vi "2021_day4_task1,2.vi"() -> ()   [LabVIEW 2021]
panel:
  out "TASK2: Winning Score (Last board)":u32
  out "TASK1: Winning Score":u32
  out "Number of Drawns":i32[](array[numeric])
  out "Winning Scores":u32[](array[numeric])
  out "5x5 Bingo numbers":i32[][][](array[numeric])
  out "array":string[](array[string])
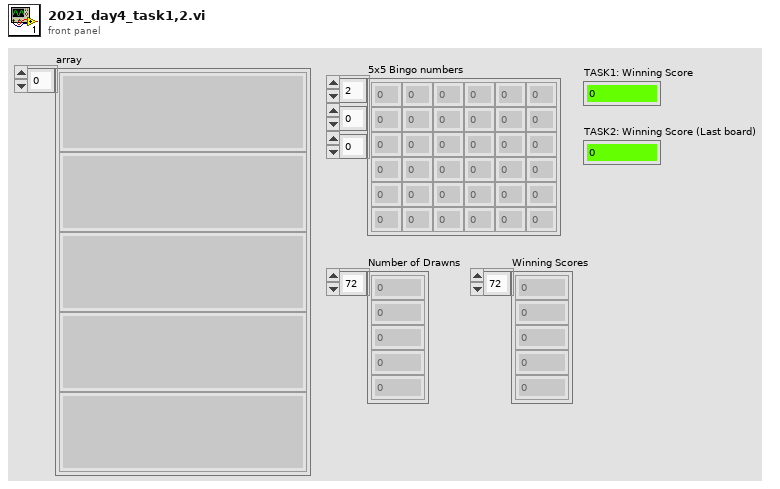
[diagram p1: front panel]
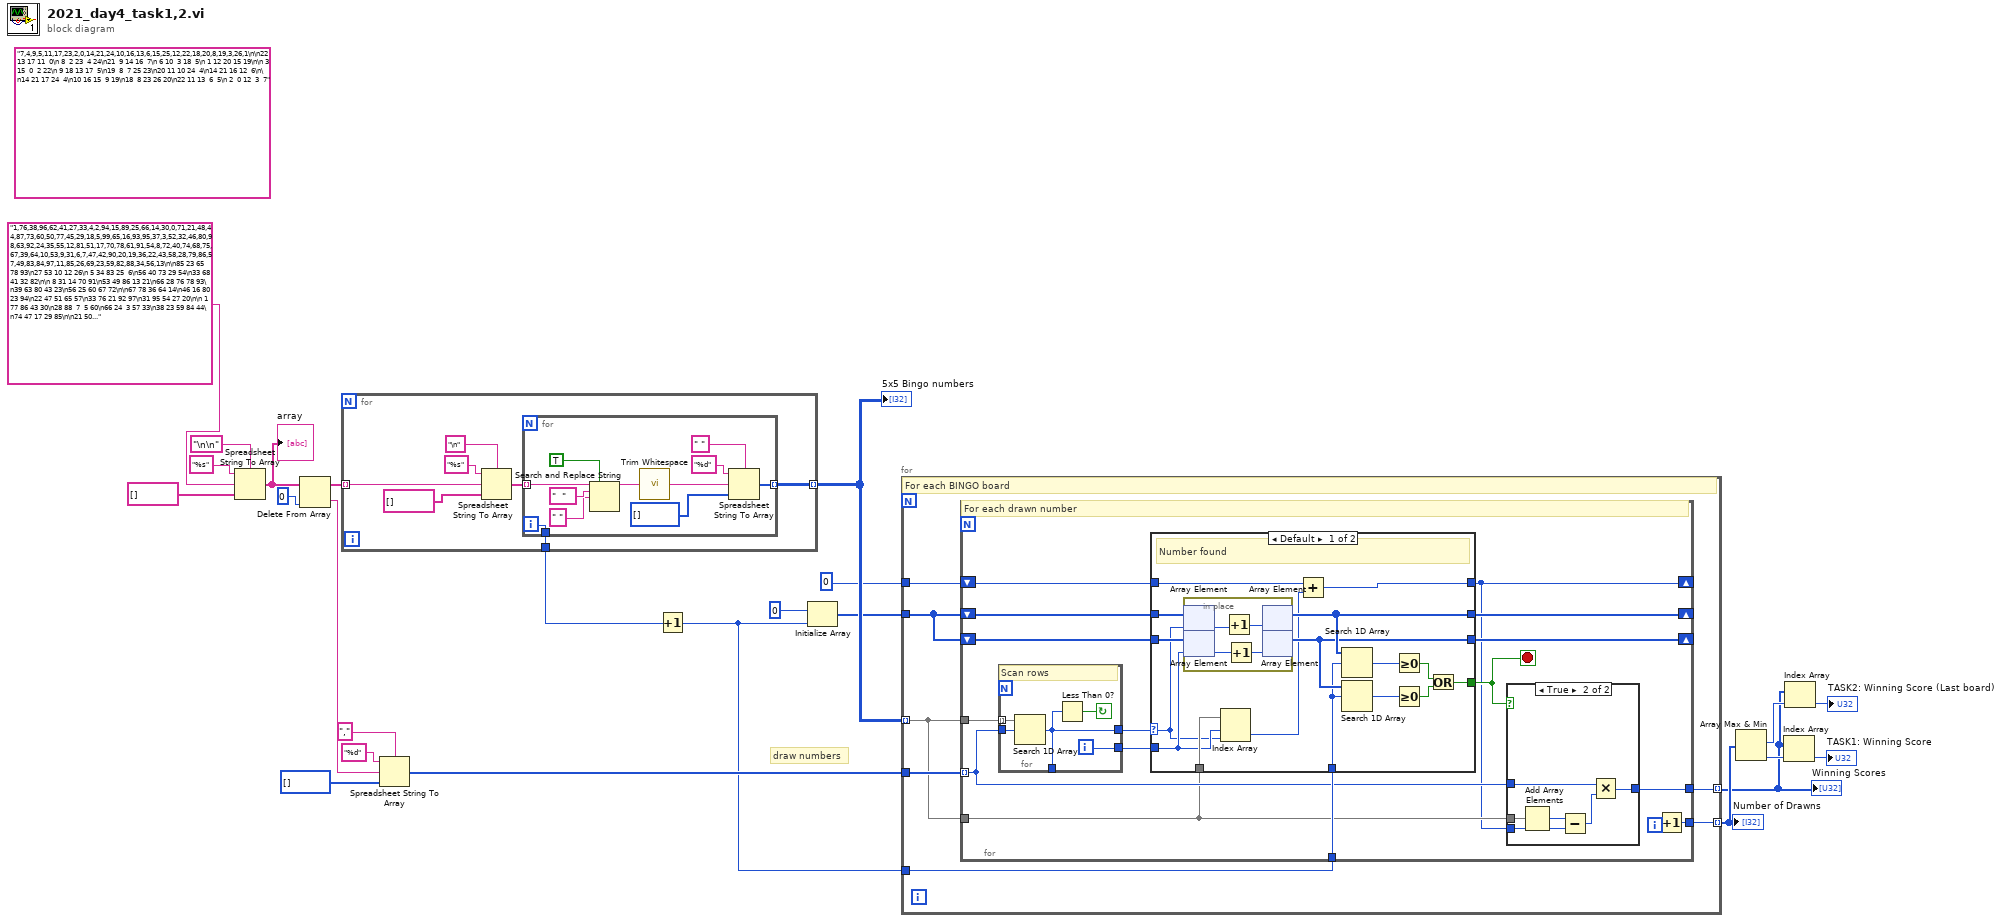
[diagram p0: block diagram]
diagram:
  (unwired) "7,4,9,5,11,17,23,2,0,14,21,24,10,16,13,6,15,25,12,22,18,20,8,19,3,26,1\n\n22 13 17 11  0\n 8  2 23  4 24\n21  9 14 16  7\n 6 10  3 18  5\n 1 12 20 15 19\n\n 3 15  0  2 22\n 9 18 13 17  5\n19  8  7 25 23\n20 11 10 24  4\n14 21 16 12  6\n\n14 21 17 24  4\n10 16 15  9 19\n18  8 23 26 20\n22 11 13  6  5\n 2  0 12  3  7"
  # "draw numbers"
  n1 = Spreadsheet String To Array(delimiter (Tab)="\n\n", format string="%s", spreadsheet string="1,76,38,96,62,41,27,33,4,2,94,15,89,25,66,14,30,0,71,21,48,44,87,73,60,50,77,45,29,18,5,99,65,16,93,95,37,3,52,32,46,80,98,63,92,24,35,55,12,81,51,17,70,78,61,91,54,8,72,40,74,68,75,67,39,64,10,53,9,31,6,7,47,42,90,20,19,36,22,43,58,28,79,86,57,49,83,84,97,11,85,26,69,23,59,82,88,34,56,13\n\n85 23 65 78 93\n27 53 10 12 26\n 5 34 83 25  6\n56 40 73 29 54\n33 68 41 32 82\n\n 8 31 14 70 91\n53 49 86 13 21\n66 28 76 78 93\n39 63 80 43 23\n56 25 60 67 72\n\n67 78 36 64 14\n46 16 80 23 94\n22 47 51 65 57\n33 76 21 92 97\n31 95 54 27 20\n\n 1 77 86 43 30\n28 88  7  5 60\n66 24  3 57 33\n38 23 59 84 44\n74 47 17 29 85\n\n21 50 86  2 70\n85 19 22 93 25\n99 38 74 30 65\n81  0 47 78 63\n34 11 51 88 64\n\n45 15 29 81 30\n75 21 88 91 49\n39 20  4 17 78\n10 12 38 11  7\n98  6 65 69 86\n\n36 20 31 44 69\n30 65 55 88 64\n74 85 82 61  5\n57 17 90 43 54\n58 83 52 23  7\n\n42 16 82 86 76\n60 26 27 59 55\n 7 53 22 78  5\n18 61 10 15 17\n28 46 14 87 77\n\n21 43 15 47 61\n24 76 28  3 27\n19 62 69 82 93\n49 29 97 74 41\n92 36 37 99 40\n\n31  4  3 62 51\n24 57 78 67 53\n13  5 76 38 55\n79  9 75 98 71\n65  1 39 18 47\n\n59  4 38 95 99\n85 68 69 93 43\n83 57 48 42 15\n47 50 80 79 90\n56 87 78 64 25\n\n21 37 14 67 95\n88 39 26 38 49\n89 83 54 77 96\n48 86 94 19 20\n43 41  8 74 58\n\n 1 36 12 90 91\n63 21 98 82 66\n39 86  7 52 77\n80 81 44 33 58\n78 30 11 51 28\n\n81 74  7 33 96\n75 60 87 47 91\n39 73 30 50 13\n 4 41  9 43 77\n34 82 72 48 12\n\n93 63 74 25 57\n29 76  9 45 70\n98 77 71 16 41\n47 54 18 14 55\n31 89 67 87 83\n\n 8 72 45 93 68\n74 26 69 94 65\n28  9 20 47 41\n46 54 21 56 22\n84 62 18 15 48\n\n20 51 81 40 69\n71 10 13 93 75\n44 86  0 95 37\n99 39 76 80 66\n14 64 49 62 27\n\n75  7 51 86 79\n43 30 61 39 16\n85 63 90 28 96\n88 78 72 31 73\n98 87 23 19 58\n\n20 95 47 97 12\n92 25 68 87 91\n37 10 78 23 63\n74 93 58 39  5\n76 51 48 72 16\n\n37 18 32 34 85\n22 31 98 42 19\n29 72 48 76 25\n47  1 21  7 53\n79 82 86 52 78\n\n20 16 47 78 92\n88 15 71 67  2\n 5 52 90 70  9\n22 49 28 82 27\n 6 19 61 73 48\n\n71 26  7 11 79\n52 30 47  1 31\n17 75 94 91 28\n81 98 23 55 21\n77 15 39 24 16\n\n 5 75 44 88 65\n89 45 23 69 19\n41 61 67 52 54\n47 38 57 12 98\n62 70 26 87 53\n\n50  4 65 77 25\n 6 21  5 27 92\n39 63 97 75 79\n60 34 87 26 74\n99 24 44 85  2\n\n13 64 38 78 21\n74 17 83 57 94\n25 39 69 53  4\n54 33 81 50 76\n42 75 19 77 26\n\n63 31 70 19 39\n38 87 15 90 75\n61 98  6 29 86\n78 62 32 11 60\n55 97 13 73 82\n\n51 63 68 84 36\n12 33 37 31  8\n18 41 34 74 23\n72 39 85 48 60\n24 19 29 88  0\n\n46 51 17 23 13\n20 93 97 99 81\n57 47 33 84 44\n28 96  2 43 56\n68 36 62 15  5\n\n81 99  5 30 10\n38 62 57  8 37\n 7 86 98  3 54\n46 82 96 15 72\n83  1 75 25 50\n\n47 57 11 61 27\n53 10 31 91 98\n76 85 55 38 23\n 6 81 67 71 70\n35 29 17 50 56\n\n24 65 15  1 89\n45 60 97 23 14\n84 56 58  5 54\n 3 72 51 46 79\n67 70 78 34 77\n\n38 11 54 23  2\n33 14 10 96 63\n43  5 36 20 30\n70 53 66 71  9\n91 90 21  7 88\n\n94 44  4 86 26\n39 70 54 50 30\n55 40 12 72 71\n68  7 66 47 91\n31 24 13  1 96\n\n79 14 40 87 68\n16 32 53 46 98\n38 95 21 89 69\n62 60 19 81 33\n70 52 28 83  0\n\n62 42 38 48 64\n61 79 78 97 98\n89  7  3 29 68\n92 76 14 67  1\n41 99 72 47 60\n\n 5 75 18 42 33\n72 61 36 31 29\n19 58  1 34 94\n54 84 92 99 38\n76 68 79 53 37\n\n14 91 37  5 98\n68 29 34 76 43\n75  0 67 33 69\n81 47 58 30 93\n88 92 42 77 54\n\n64 24 28 54 53\n72 68  3 73  4\n83  6 59 66 94\n87 80 55 20 16\n13 82 74 31 70\n\n63 92 71  0 83\n98 40 50 55  2\n88  5 85 30 23\n10 75 81 58 68\n51 31 14 89  1\n\n67 93 94 54 53\n38 71 34 40 24\n31 63 30 99 75\n 4 57 86 19 70\n60 49 87 68 74\n\n56 94 79 53  7\n24 12 19  6 99\n82 51 41 46 43\n17 49 52 78 55\n75 48 61 70 87\n\n14 55 32 21 31\n88 83 23 44  4\n 1 77 45 90 85\n46 81 51 27 62\n60 24 29 18  0\n\n95 92 91 27 26\n22 43 45 64 62\n83 23 25 85 94\n84 53 72 28 20\n75 60 52 18 73\n\n95 41  7 21 32\n58 65 16 56 97\n68 25 91 83 24\n66 89 15 55  6\n 2 30 84 10 90\n\n58 86 44 19 74\n57 89 17  6 83\n77 35 60 32 13\n97 63 62 28 76\n55 31 11  0 52\n\n33 39 59 42 45\n61 50 92  9 79\n15  0 28  5 72\n91 24 21 29 87\n86 76 43 31 93\n\n63 11 86 45 85\n96 74 66 93 32\n95 30 99 23 18\n69 97 48 15  1\n42 87 47 83 80\n\n93  5 40 64  2\n44 51 15 54 83\n69 77 90 58 11\n 0 48 43 30 55\n25 72 38 73 52\n\n89 58 71 68 15\n23 65  9 36 74\n21 29 42 79 98\n55 47 33 39 28\n16 75 91 69 57\n\n13 79 12 71  2\n60 94 99 43 82\n84 89 29 91 87\n74 80 25 32 21\n70 14 68 92 11\n\n78  1 16 51 87\n58 94 59 15 43\n79 41 50 47 39\n53 37  9 28 72\n34 63 89 35 18\n\n31 67 70 42 43\n60  2 89 49 22\n56 17 81 24 74\n20 65  1 96 51\n68  7  0 38 25\n\n59 14 29 53 19\n 9  2 11 33 44\n81  6 10 47 58\n20 34 62 55 40\n71 38 69 45 78\n\n59 36 70 42 21\n 3 16 49 79 98\n74 25  8 84 19\n61 80 47 65 64\n91 62 52  9 40\n\n 1 85 63  7  2\n 0 20 61 26 77\n99 37 74 42 76\n25 94 19 78 60\n79 72 95 22 11\n\n51 21 79 76 32\n55 23 69 19 61\n71 54 94 47 92\n 5 64  6 68 16\n91 81  9 99 30\n\n61 69 82 86 68\n66 81 28 38 36\n26 29 31 11  8\n72 51 12 95 63\n18 30 88 17 32\n\n34  8 14 42 67\n66 79 65 20 52\n37 87 74 24  3\n59 54 21 32 89\n31  4 62 76 30\n\n11 93  8 92 55\n38 72 99  3 83\n12 75  0 41 46\n17 25  5 39 48\n14 18 86 29 84\n\n 6 20 41 51 48\n 5 67 30 24 47\n 3  8 92 22 39\n 4 56 36 31 75\n 2 45 85 81 96\n\n47 43 72 22  3\n19 87 53 12 60\n29 40 56 68 18\n66 97 70 33 39\n85 37  0 90 98\n\n61 35 81 84 94\n11  1 58 45 77\n 6 99 67 36 43\n 5  7  0 87 80\n44 78 39 70 20\n\n58 34 49 29 75\n17 15 28 23 84\n59 25 92 48  0\n20 81 47  3 71\n68 60  5 22 87\n\n90 32 41 39  6\n36 78 67 24 50\n55 72 52 75 44\n87 15 92 31 58\n83 89 68 19 43\n\n99 44 53 68 25\n71 67 16 19 36\n35 58 14 86 48\n88 18 61 24 23\n87  9 91 37 15\n\n37  5 63 68 28\n41 50 76 99 64\n34 92 78 94 71\n11 96 97 42 58\n33 45  0 93 48\n\n33 68  9 12 81\n60 98 28  8 99\n14 17  6 82 15\n57 69 43 38 29\n47 84 76 22 18\n\n79 70 92 38 47\n12 82 98 46  0\n76 15 53 59 97\n18 52 49 29 96\n44 64 68 89 24\n\n95 14 17 27 42\n55 43 57 29 25\n34 73 86 50 16\n69 37 75 63 39\n78 79  3  4 30\n\n27 31 15 92 46\n36 23 72 40 50\n51 99 55 89 21\n12 70 84 63 85\n78 88 77 75  0\n\n15 67 40 39 28\n 9 79 22 52 75\n96 65 86 98 14\n97 87 44 84 68\n36 26 89 43 27\n\n79 59 48 27 36\n85 92 93 76 24\n 2 25  7 42 90\n23 29 74 35 86\n58 60 31 75 57\n\n10 43 83 75  8\n88 12 38 30  9\n60 67 59 76  6\n55 45 74 34 25\n97 49 65 96 69\n\n59 86 15  3 19\n89  4 74 61 23\n52 98  8 79 39\n95 17 22 14 51\n50 18 94 30 84\n\n19 63 58 72 67\n35 93 29 91  0\n39 26 43 84 21\n70 42  2 53 12\n59 99  8  1 86\n\n23 86 34 22 65\n71 10 16 50 91\n66 89 49 81 43\n40  7 26 75 61\n62 59  2 46 95\n\n24 21  0 49 25\n92 42 48 12  7\n81 93 59 68  3\n14 23 63 39 29\n35 43  6 44 89\n\n67 74 95 34 10\n39 90 59 44 51\n17 16 97 24 62\n20 54 76 63 88\n87 66 14 78 82\n\n96 86 67 59 79\n66  3 30 77 71\n 2 91 99 82 31\n48 65 75 98 53\n63 54 64 76  1\n\n85 96 40 98 24\n16 20 10 23 17\n79 59 53 42 65\n67  2  5 80 75\n62 38 19 74 73\n\n43 10 79 92  8\n52 36  4  5 67\n56 29 33 24 97\n85 17 53 75 65\n62 64  1 21 83\n\n93 92 79 17 12\n40 88  6 82 34\n90 96 53 25 43\n14 62 54 10 39\n49 68 41 16 44\n\n67 99 24 58 76\n43 53 59 54 51\n47  6 61  8  2\n80 68 90 14  4\n29 46 94 89 50\n\n14 45 19 33 43\n 6 55  4 31 80\n51  2 69 68 61\n71 70 79 91 93\n66 18 54 13 87\n\n 8 45 61 54 30\n85 16 19 82 37\n56 39 11 47  4\n74 70 10 60 91\n21 63 95 53 72\n\n71 21 63 86 27\n53 52 40 23 81\n 2 47 92 68 15\n46 45 31  8  1\n34 80 37 11 69\n\n96  0 15 90 66\n65 43 92 83 18\n 3 47 19  8 32\n71 26 42 34 28\n62 99 55  5 12\n\n37 99 30 21  3\n63 18 68 47 27\n57  0 65 85 20\n 7 58 40 92 43\n15 19  5  4 53\n\n46 16 45 95 68\n 6 44 31 47 73\n84 82 71 75 94\n26 25 17 32 49\n18 96 13 58  9\n\n71 36 13 68 10\n84  7 60 79 41\n 1 83 43 81 97\n90 53 80 19 38\n48 25 32 42 29\n\n37 68 86 44 78\n87 67 77 70 60\n45 34 27 15 47\n12 21 13 55 26\n81 41 63 40 74\n\n24 50 93 94 57\n99  4 56  5 28\n42 31 22  6 76\n90 89 16 49 59\n 9  7 43 71 54\n\n69 75 94 38 46\n52 64 50 72 42\n76 63 13 60 10\n99 80 43 33 17\n25 31  4 89 22\n\n88 57 22 66 34\n85 16 87 95 59\n73  2 46  5 29\n25 69 53  6 14\n96 77 19 91 43\n\n46 99 52 47 76\n89 53 24 13 59\n45  5  1 30 19\n68 25 22 10 73\n42 27 31  0 94\n\n42 44 98 89 87\n65 10 80 56 41\n 3 35 95 48 43\n85 97 83 12 94\n50 38 93 47 17\n\n16 73 18 81 89\n 6 48 54 93 19\n35 52 88 49 31\n43 79 83 14 28\n50 62 98 26 22\n\n38 47  7 20 35\n45 76 63 96 24\n98 53  2 87 80\n83 86 92 48  1\n73 60 26 94  6\n\n80 50 29 53 92\n66 90 79 98 46\n40 21 58 38 60\n35 13 72 28  6\n48 76 51 96 12\n\n79 80 24 37 51\n86 70  1 22 71\n52 69 10 83 13\n12 40  3  0 30\n46 50 48 76  5\n" ("format string"), array type (2D Dbl)=string[] []) -> (array=w21:string[])
  "array" <- w21
  n2 = Delete From Array(array=w21, index=0) -> (deleted portion=w17:string, array with subset deleted=w14:string[])  [unwired: 1 in]
  n3 = for {
    tunnel: w14 -> [w30] mode=indexing
    tunnel: [w31] -> w13 mode=indexing
    tunnel: [w25] -> w10
    n4 = Spreadsheet String To Array(delimiter (Tab)="\n", format string="%s", spreadsheet string=w30, array type (2D Dbl)=string[] []) -> (array=w26:string[])
    n5 = for {
      tunnel: [w40] -> w31 mode=indexing
      tunnel: w26 -> [w39] mode=indexing
      tunnel: [w32] -> w25
      i -> [w32]
      n6 = Search and Replace String(replace all?=TRUE ("replace all? (F)"), input string=w39, search string="  " ("delimiter (Tab)"), replace string=" " ("delimiter (Tab)")) -> (result string=w34:string)  [unwired: 4 in, 3 out]
      n7 = call <vilib>:"Trim Whitespace.vi"("string"=w34) -> ("trimmed string"=w33:string)  [unwired: 1 in]
      n8 = Spreadsheet String To Array(delimiter (Tab)=" ", format string="%d", spreadsheet string=w33, array type (2D Dbl)=i32[] []) -> (array=w40:i32[])
    }
  }
  "5x5 Bingo numbers" <- w13
  n9 = Spreadsheet String To Array(delimiter (Tab)=",", format string="%d", spreadsheet string=w17, array type (2D Dbl)=u32[] []) -> (array=w15:u32[])
  n10 = Increment(x=w10) -> (x+1=w9:i32)
  n11 = Initialize Array(u32 0, w9) -> (w11:u32[])
  n12 = for {
    tunnel: w15 -> [w49]
    tunnel: w13 -> [w46] mode=indexing
    tunnel: w11 -> [w48]
    tunnel: w9 -> [w47]
    tunnel: [w45] -> w2 mode=indexing
    tunnel: [w44] -> w3 mode=indexing
    tunnel: u32 0 -> [w43]
    # "For each BINGO board"
    n13 = for {
      tunnel: w49 -> [w57] mode=indexing
      tunnel: w46 -> [w65]
      shift-right: [w62] -> _
      shift-left: w48 -> [w64]
      shift-right: [w61] -> _
      shift-left: w48 -> [w63]
      tunnel: w47 -> [w58]
      tunnel: w46 -> [w55]
      tunnel: [w54] -> w45
      tunnel: [w52] -> w44
      shift-right: [w50] -> _
      shift-left: w43 -> [w51]
      i -> [w53]
      stop <- w56 stop-if-true
      # "For each drawn number"
      n14 = for {
        tunnel: w65 -> [w93] mode=indexing
        tunnel: w57 -> [w92]
        tunnel: [w91] -> w59
        tunnel: [w89] -> _
        tunnel: [w89] -> w60
        i -> [w91]
        stop <- w90 continue-if-true
        # "Scan rows"
        n15 = Search 1D Array(1D array=w93, element=w92) -> (index of element=w89:i32)  [unwired: 1 in]
        n16 = Less Than 0?(x=w89) -> (x < 0?=w90:bool)
      }
      n17 = case shown="Default" w60 {
        selector: w60 -> [w66 _]
        tunnel: w64 -> [w81 w88]
        tunnel: w63 -> [w80 w87]
        tunnel: [w79 w88] -> w62
        tunnel: [w78 w87] -> w61
        tunnel: w59 -> [w67 _]
        tunnel: w58 -> [w77 _]
        tunnel: [w75 _] -> w56
        tunnel: w55 -> [w74 _]
        tunnel: [w69 w86] -> w50
        tunnel: w51 -> [w70 w86]
        frame Default {
          # "Number found"
          n18 = in-place {
            n19 = in-place-array #1(w81, w66) -> (w85:u32)
            n20 = in-place-array #2(w80, w67) -> (w83:u32)
            n21 = Increment(x=w85) -> (x+1=w84:u32)
            n22 = Increment(x=w83) -> (x+1=w82:u32)
            n23 = in-place-array #1(w84) -> (w79:u32[])  [unwired: 1 out]
            n24 = in-place-array #2(w82) -> (w78:u32[])  [unwired: 1 out]
          }
          n25 = Index Array(array=w74, index (row)=w67, index (col)=w66) -> (element=w68:i32)
          n26 = Add(x=w70, y=w68) -> (x+y=w69:u32)
          n27 = Search 1D Array(1D array=w79, element=w77) -> (index of element=w71:i32)  [unwired: 1 in]
          n28 = Search 1D Array(1D array=w78, element=w77) -> (index of element=w73:i32)  [unwired: 1 in]
          n29 = Greater Or Equal To 0?(x=w71) -> (x >= 0?=w76:bool)
          n30 = Greater Or Equal To 0?(x=w73) -> (x >= 0?=w72:bool)
          n31 = Or(x=w76, y=w72) -> (x .or. y?=w75:bool)
        }
        frame -1 {
          # "Number not found"
        }
      }
      n32 = case shown="True" w56 {
        tunnel: w57 -> [_ w99]
        tunnel: w55 -> [_ w98]
        tunnel: w50 -> [_ w96]
        tunnel: [_ w94] -> w54
        frame False {
        }
        frame True {
          n33 = Add Array Elements(numeric array=w98) -> (sum=w97:i32)
          n34 = Subtract(x=w97, y=w96) -> (x-y=w95:u32)
          n35 = Multiply(x=w99, y=w95) -> (x*y=w94:u32)
        }
      }
      n36 = Increment(x=w53) -> (x+1=w52:i32)
    }
  }
  "Winning Scores" <- w2
  "Number of Drawns" <- w3
  n37 = Array Max & Min(array=w3) -> (max index (indices)=w4:i32, min index (indices)=w7:i32)  [unwired: 2 out]
  n38 = Index Array(array=w2, index=w7) -> (element=→"TASK1: Winning Score":u32)
  n39 = Index Array(array=w2, index=w4) -> (element=→"TASK2: Winning Score (Last board)":u32)
